vi "Merge DCIMG files.vi"(5 "Frames to Skip":u32, 6 "Horizontal Flip":bool[](array[boolean]), 7 "Vertical Flip":bool[](array[boolean]), 8 "error in (no error)":errorcluster, 9 "Channel 3 Right?":bool, 10 "DCIMG Paths (2 to 4)":path[](array[path]), 11 "TIFF in":refnum<class "TIFF.lvclass">) -> (0 "error out":errorcluster, 3 "TIFF out":refnum<class "TIFF.lvclass">)   [LabVIEW 2022 SP3, in "BinaryTIFF.lvlib" / "TIFF.lvclass"]
uses:
  TIFF.lvclass
  TIFF.lvclass/TIFF.ctl
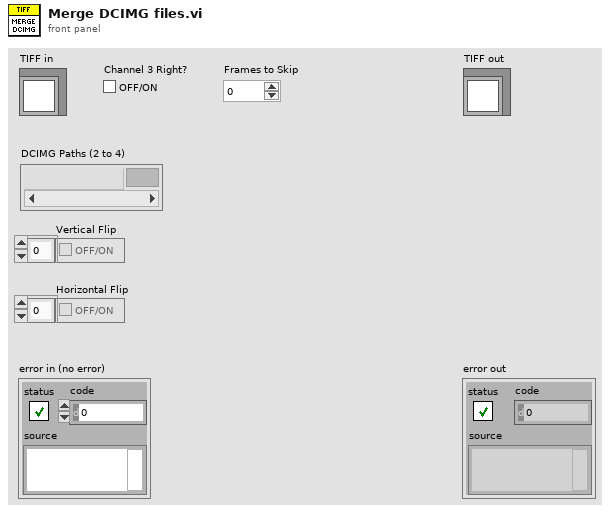
[diagram p1: front panel]
types:
  T1 = typedef "Camera Type.ctl" = enum16{"Hamamatsu", "Andor", "Photometrics"}
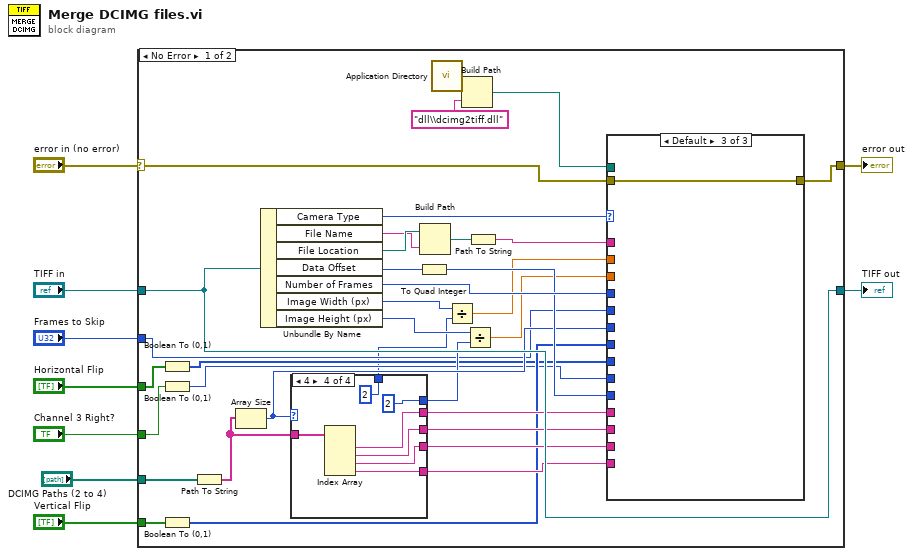
[diagram p0: block diagram]
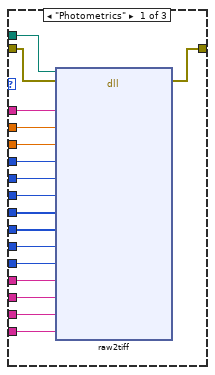
[diagram p2: hidden frame]
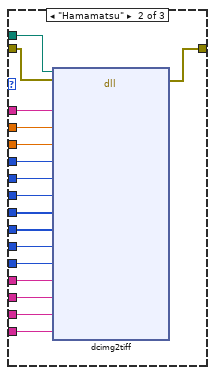
[diagram p3: hidden frame]
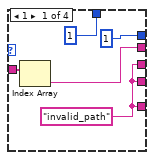
[diagram p4: hidden frame]
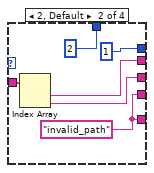
[diagram p5: hidden frame]
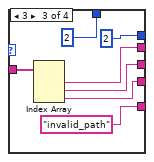
[diagram p6: hidden frame]
diagram:
  n1 = case shown="No Error" "error in (no error)" {
    selector: "error in (no error)" -> [w13 w105]
    tunnel: [w10 w105] -> w8
    tunnel: [w43 w104] -> w6
    tunnel: "TIFF in" -> [w43 w104]
    tunnel: "Horizontal Flip" -> [w23 _]
    tunnel: "Vertical Flip" -> [w24 _]
    tunnel: "Channel 3 Right?" -> [w22 _]
    tunnel: "Frames to Skip" -> [w18 _]
    tunnel: "DCIMG Paths (2 to 4)" -> [w12 _]
    frame No Error {
      n2 = Boolean To (0,1)(Boolean=w23) -> (0, 1=w20:i16[])
      n3 = Boolean To (0,1)(Boolean=w22) -> (0, 1=w19:i16)
      n4 = Boolean To (0,1)(Boolean=w24) -> (0, 1=w21:i16[])
      n5 = Path To String(path=w12) -> (string=w33:string[])
      n6 = Array Size(array=w33) -> (size(s)=w28:i32)
      n7 = Unbundle By Name(w43) -> ("Camera Type"=w11:T1, "File Name"=w41:string, "File Location"=w42:path, "Data Offset"=w38:u64, "Number of Frames"=w37:u32, "Image Width (px)"=w34:u32, "Image Height (px)"=w27:u32)
      n8 = case shown="4" w28 {
        tunnel: w33 -> [w83 w89 w96 w103]
        tunnel: [w82 w88 w95 w102] -> w32
        tunnel: [w79 w87 w94 w101] -> w31
        tunnel: [w79 w86 w92 w100] -> w30
        tunnel: [w79 w86 "invalid_path" ("DCIMG Path 1") w99] -> w29
        tunnel: [u32 1 ("y") u32 1 ("y") u32 2 ("y") u32 2 ("y")] -> w25
        tunnel: [u32 1 ("y") u32 2 ("y") u32 2 ("y") u32 2 ("y")] -> w17
        frame 1 {
          w79 = "invalid_path" ("DCIMG Path 1")
          n9 = Index Array(array=w83) -> (element=w82:string)  [unwired: 1 in]
        }
        frame 2, Default {
          w86 = "invalid_path" ("DCIMG Path 1")
          n10 = Index Array(array=w89) -> (element #1=w88:string, element #2=w87:string)  [unwired: 2 in]
        }
        frame 3 {
          n11 = Index Array(array=w96) -> (element #1=w95:string, element #2=w94:string, element #3=w92:string)  [unwired: 3 in]
        }
        frame 4 {
          n12 = Index Array(array=w103) -> (element #1=w102:string, element #2=w101:string, element #3=w100:string, element #4=w99:string)  [unwired: 4 in]
        }
      }
      n13 = To Quad Integer(1:w38) -> (0:w36:i64)
      n14 = Build Path(base path=w42, name or relative path=w41) -> (appended path=w40:path)
      n15 = call <vilib>:"Application Directory.vi"() -> ("Application Directory"=w15:path)
      n16 = Divide(x=w34, y=w17) -> (x/y=w35:dbl)
      n17 = Build Path(base path=w15, name or relative path="dll\\dcimg2tiff.dll") -> (appended path=w14:path)
      n18 = Divide(x=w27, y=w25) -> (x/y=w26:dbl)
      n19 = Path To String(path=w40) -> (string=w39:string)
      n20 = case shown="Default" w11 {
        tunnel: w39 -> [w57 w77 _]
        tunnel: w13 -> [w59 w76 w78]
        tunnel: [w58 w75 w78] -> w10
        tunnel: w37 -> [w54 w74 _]
        tunnel: w36 -> [w48 w73 _]
        tunnel: w35 -> [w56 w72 _]
        tunnel: w32 -> [w47 w71 _]
        tunnel: w31 -> [w46 w70 _]
        tunnel: w30 -> [w45 w69 _]
        tunnel: w29 -> [w44 w68 _]
        tunnel: w28 -> [w52 w67 _]
        tunnel: w26 -> [w55 w66 _]
        tunnel: w21 -> [w51 w65 _]
        tunnel: w20 -> [w50 w64 _]
        tunnel: w19 -> [w49 w63 _]
        tunnel: w18 -> [w53 w62 _]
        tunnel: w14 -> [w60 w61 _]
        frame "Photometrics" {
          n21 = dll-call lib="?" fn="raw2tiff"(path in=w60, error in=w59, "TIFF Path"=w57, "Frame Width"=w56, "Frame Height"=w55, "N Frames"=w54, "Frames to Skip"=w53, "N Channels"=w52, "Vertical Flip"=w51, "Horizontal Flip"=w50, "Channel 3 Right?"=w49, "TIFF Offset"=w48, "DCIMG Path 1"=w47, "DCIMG Path 2"=w46, "DCIMG Path 3 (opt.)"=w45, "DCIMG Path 4 (opt.)"=w44) -> (error out=w58:errorcluster)  [unwired: 16 in, 1 out]
        }
        frame "Hamamatsu" {
          n22 = dll-call lib="?" fn="dcimg2tiff"(path in=w61, error in=w76, "TIFF Path"=w77, "Frame Width"=w72, "Frame Height"=w66, "N Frames"=w74, "Frames to Skip"=w62, "N Channels"=w67, "Vertical Flip"=w65, "Horizontal Flip"=w64, "Channel 3 Right?"=w63, "TIFF Offset"=w73, "DCIMG Path 1"=w71, "DCIMG Path 2"=w70, "DCIMG Path 3 (opt.)"=w69, "DCIMG Path 4 (opt.)"=w68) -> (error out=w75:errorcluster)  [unwired: 16 in, 1 out]
        }
        frame Default {
        }
      }
    }
    frame Error {
    }
  }
  "error out" <- w8
  "TIFF out" <- w6
